vi "Switch Configuration - Filter to Mux.vi"(8 "error in (no error)":errorcluster, 11 "Switch Config UI Data In":T1 {"Switch Config Page Item Ref" format="%.0x"}) -> (0 "error out":errorcluster, 3 "Switch Config UI Data Out":T1 {"Switch Config Page Item Ref" format="%.0x"})   [LabVIEW 2015, in "DMM-SWITCH-ScanList System Explorer.lvlib"]
doc: "Filters supported Mux Topologies from al Switch (Matrix and Mux) Supported Topologies. Supported Switch Topologies come from the NI-Switch Type Def Topology Control. This Type Def should be updated with more supported models in future versions of NI-Switch."
uses:
  DMM-SWITCH-ScanList System Explorer.lvlib
  Configuration Controls/Switch Config VI UI Data.ctl
  Configuration Controls/Switch Config VI UI Ctrl Values.ctl
  Configuration Controls/Switch Config VI UI Ctrl References.ctl
  <instrlib>/niSwitch/niSwitch.LLB/niSwitch Topologies.ctl
  <vilib>/NI Veristand/Custom Device API/Custom Device Item Ref.ctl
  <vilib>/NI Veristand/Custom Device API/Custom Device API.lvlib
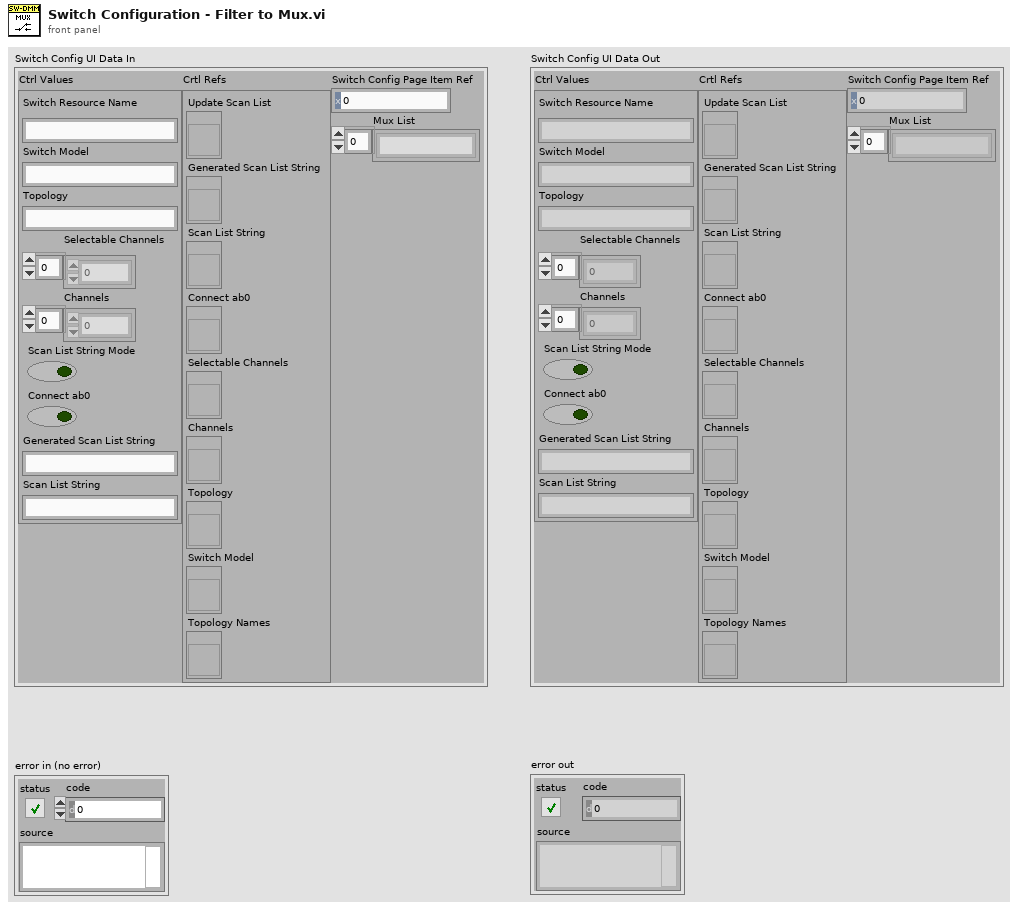
[diagram p1: front panel]
types:
  T1 = typedef "DMM-SWITCH-ScanList System Explorer.lvlib/Switch Config VI UI Data.ctl" = cluster{"Ctrl Values":T2, "Crtl Refs":T3, "Switch Config Page Item Ref":T4, "Mux List":string[]}
  T2 = typedef "DMM-SWITCH-ScanList System Explorer.lvlib/Switch Config VI UI Ctrl Values.ctl" = cluster{"Switch Resource Name":string, "Switch Model":string, "Topology":string, "Selectable Channels":i32[], "Channels":i32[], "Scan List String Mode":bool, "Connect ab0":bool, "Generated Scan List String":string, "Scan List String":string}
  T3 = typedef "DMM-SWITCH-ScanList System Explorer.lvlib/Switch Config VI UI Ctrl References.ctl" = cluster{"Update Scan List":refnum<vi>, "Generated Scan List String":refnum<vi>, "Scan List String":refnum<vi>, "Connect ab0":refnum<vi>, "Selectable Channels":refnum<vi>, "Channels":refnum<vi>, "Topology":refnum<vi>, "Switch Model":refnum<vi>, "Topology Names":refnum<vi>}
  T4 = typedef "Custom Device API.lvlib/Custom Device Item Ref.ctl" = u64
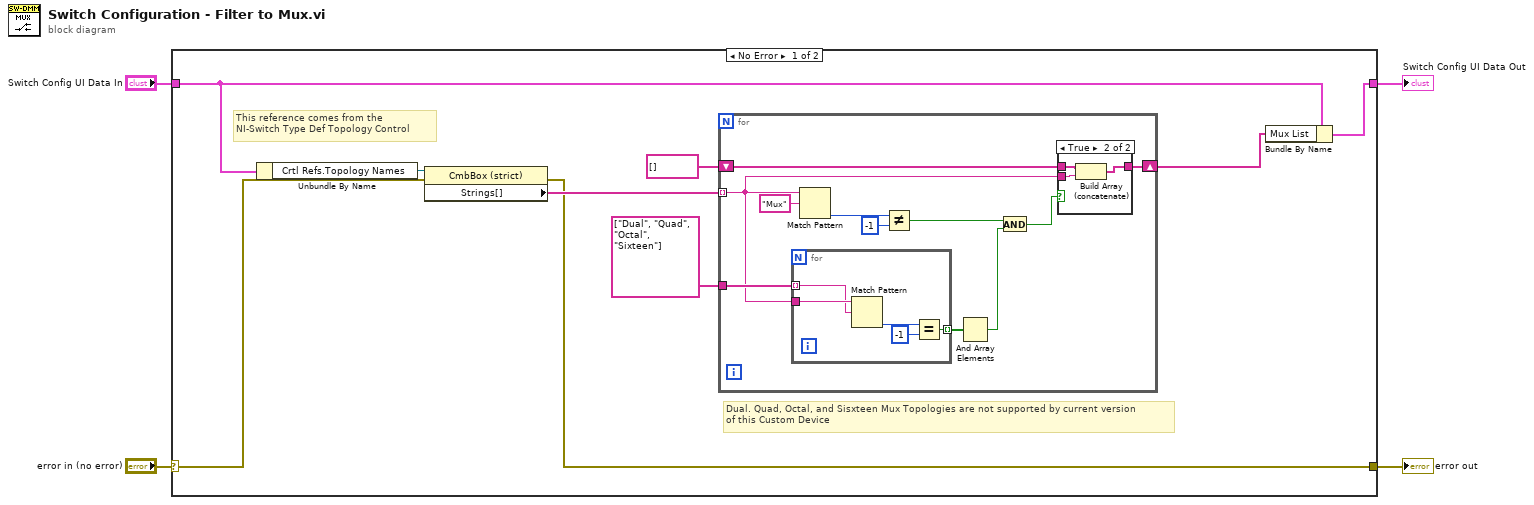
[diagram p0: block diagram]
diagram:
  n1 = case shown="No Error" "error in (no error)" {
    selector: "error in (no error)" -> [w10 w35]
    tunnel: [w9 w35] -> w3
    tunnel: "Switch Config UI Data In" -> [w7 w34]
    tunnel: [w5 w34] -> w1
    frame No Error {
      # "This reference comes from the \nNI-Switch Type Def Topology Control"
      # "Dual. Quad, Octal, and Sisxteen Mux Topologies are not supported by current version\nof this Custom Device"
      n2 = Unbundle By Name(w7) -> ("Crtl Refs.Topology Names"=w8:refnum<vi>)
      n3 = property class="CmbBox (strict)"(reference=w8, error in=w10) -> (error out=w9:errorcluster, "Strings[]"=w13:string[])  [unwired: 1 out]
      n4 = for {
        tunnel: w13 -> [w18] mode=indexing
        shift-right: [w21] -> w6
        shift-left: string[] [] ("Strings []") -> [w22]
        tunnel: string[] ["Dual", "Quad", "Octal", "Sixteen"] -> [w19]
        n5 = for {
          tunnel: w19 -> [w26] mode=indexing
          tunnel: w18 -> [w27]
          tunnel: [w25] -> w17 mode=indexing
          n6 = Match Pattern(string=w27, regular expression=w26) -> (offset past match=w28:i32)  [unwired: 1 in, 3 out]
          n7 = Equal?(x=w28, y=-1) -> (x = y?=w25:bool)
        }
        n8 = Match Pattern(string=w18, regular expression="Mux") -> (offset past match=w23:i32)  [unwired: 1 in, 3 out]
        n9 = Not Equal?(x=w23, y=-1) -> (x != y?=w16:bool)
        n10 = And Array Elements(Boolean array=w17) -> (logical AND=w15:bool)
        n11 = And(x=w16, y=w15) -> (x .and. y?=w14:bool)
        n12 = case shown="True" w14 {
          tunnel: w22 -> [w30 w33]
          tunnel: w18 -> [_ w32]
          tunnel: [w30 w31] -> w21
          frame False {
          }
          frame True {
            n13 = Build Array (concatenate)(w33, w32) -> (w31:string[])
          }
        }
      }
      n14 = Bundle By Name(cluster=w7, "Mux List"=w6) -> (w5:T1)
    }
    frame Error {
    }
  }
  "error out" <- w3
  "Switch Config UI Data Out" <- w1
